vi "String_SpectralStabilitySettings.vi"(8 "Duration/Times":bool, 9 "Measurement Number":u32, 10 "Duration":dbl[unit], 11 "Periodic Time":dbl[unit]) -> (3 "String":string)   [LabVIEW 2020]
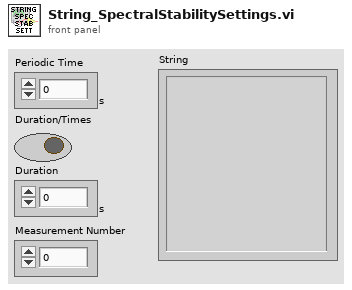
[diagram p1: front panel]
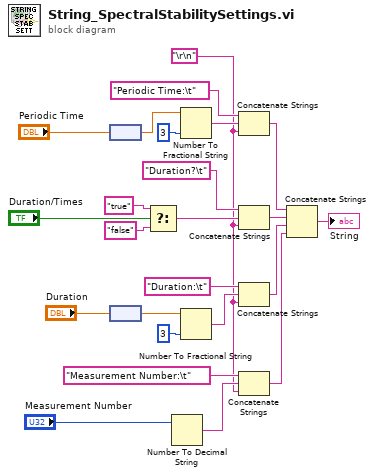
[diagram p0: block diagram]
diagram:
  w6 = "\r\n"
  n1 = node("Periodic Time") -> (w15:dbl)
  n2 = node("Duration") -> (w12:dbl)
  n3 = Select(t="true", s="Duration/Times", f="false") -> (s? t:f=w16:string)
  n4 = Number To Decimal String(number="Measurement Number") -> (decimal integer string=w7:string)  [unwired: 1 in]
  n5 = Number To Fractional String(number=w15, precision (6)=i16 3) -> (F-format string=w21:string)  [unwired: 2 in]
  n6 = Number To Fractional String(number=w12, precision (6)=i16 3) -> (F-format string=w11:string)  [unwired: 2 in]
  n7 = Concatenate Strings("Periodic Time:\t", w21, w6) -> (w5:string)
  n8 = Concatenate Strings("Duration?\t", w16, w6) -> (w4:string)
  n9 = Concatenate Strings("Duration:\t", w11, w6) -> (w3:string)
  n10 = Concatenate Strings("Measurement Number:\t", w7, w6) -> (w2:string)
  n11 = Concatenate Strings(w5, w4, w3, w2) -> (→"String":string)
